vi "GetVariableIDs_Example.vi"(8 "Fehler (Eingang, kein Fehler)":errorcluster) -> (0 "Fehler (Ausgang)":errorcluster, 3 "VariableArray out":T1)   [LabVIEW 2016]
uses:
  VariableArray.ctl
  VariableInfo.ctl
  girpcutil_params.ctl
panel:
  out "State":string
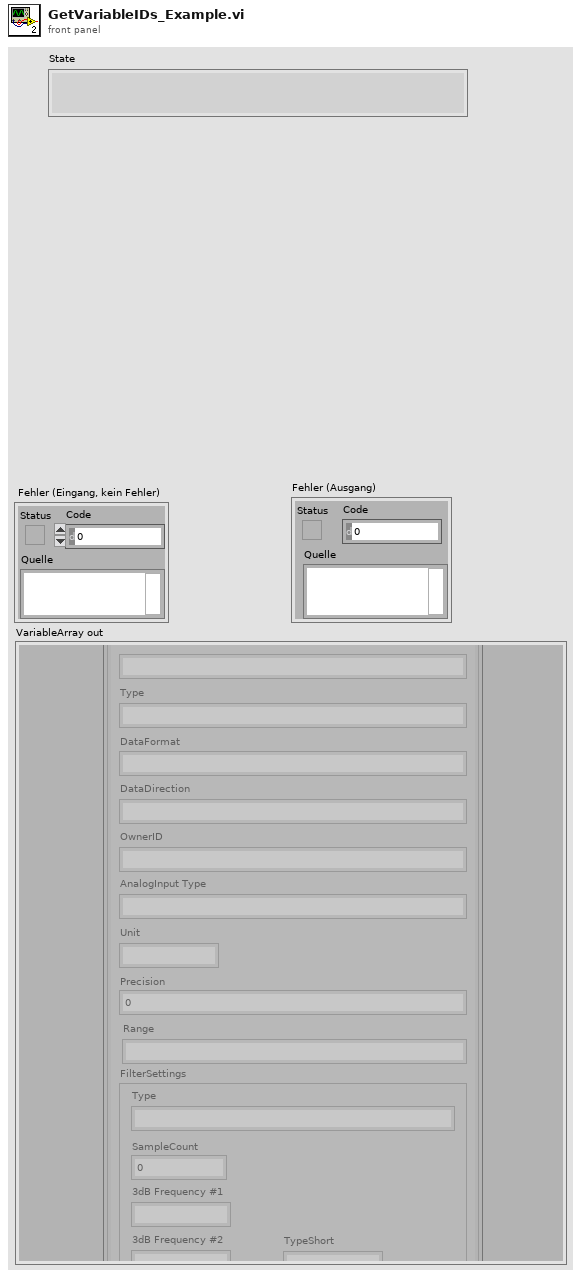
[diagram p1: front panel]
types:
  T1 = typedef "VariableArray.ctl" = cluster{"Array":T2[]}
  T2 = typedef "VariableInfo.ctl" = cluster{"Name":string, "ID":string, "Type":string, "DataFormat":string, "DataDirection":string, "OwnerID":string, "AnalogInput Type":string, "Unit":string, "Precision":dbl, "Range":string, "FilterSettings":cluster{"Type":string, "SampleCount":i64, "3dB Frequency #1":string, "3dB Frequency #2":string, "TypeShort":string}}
  T3 = typedef "girpcutil_params.ctl" = cluster{"ConnectionHandle":i32, "DLL-Handle":cluster{"DLL Path":path, "Is32Bit":bool}}
  T4 = enum16{"Bool", "Snippet", "Struct", "Int64", "Int32", "Float", "Double", "String"}
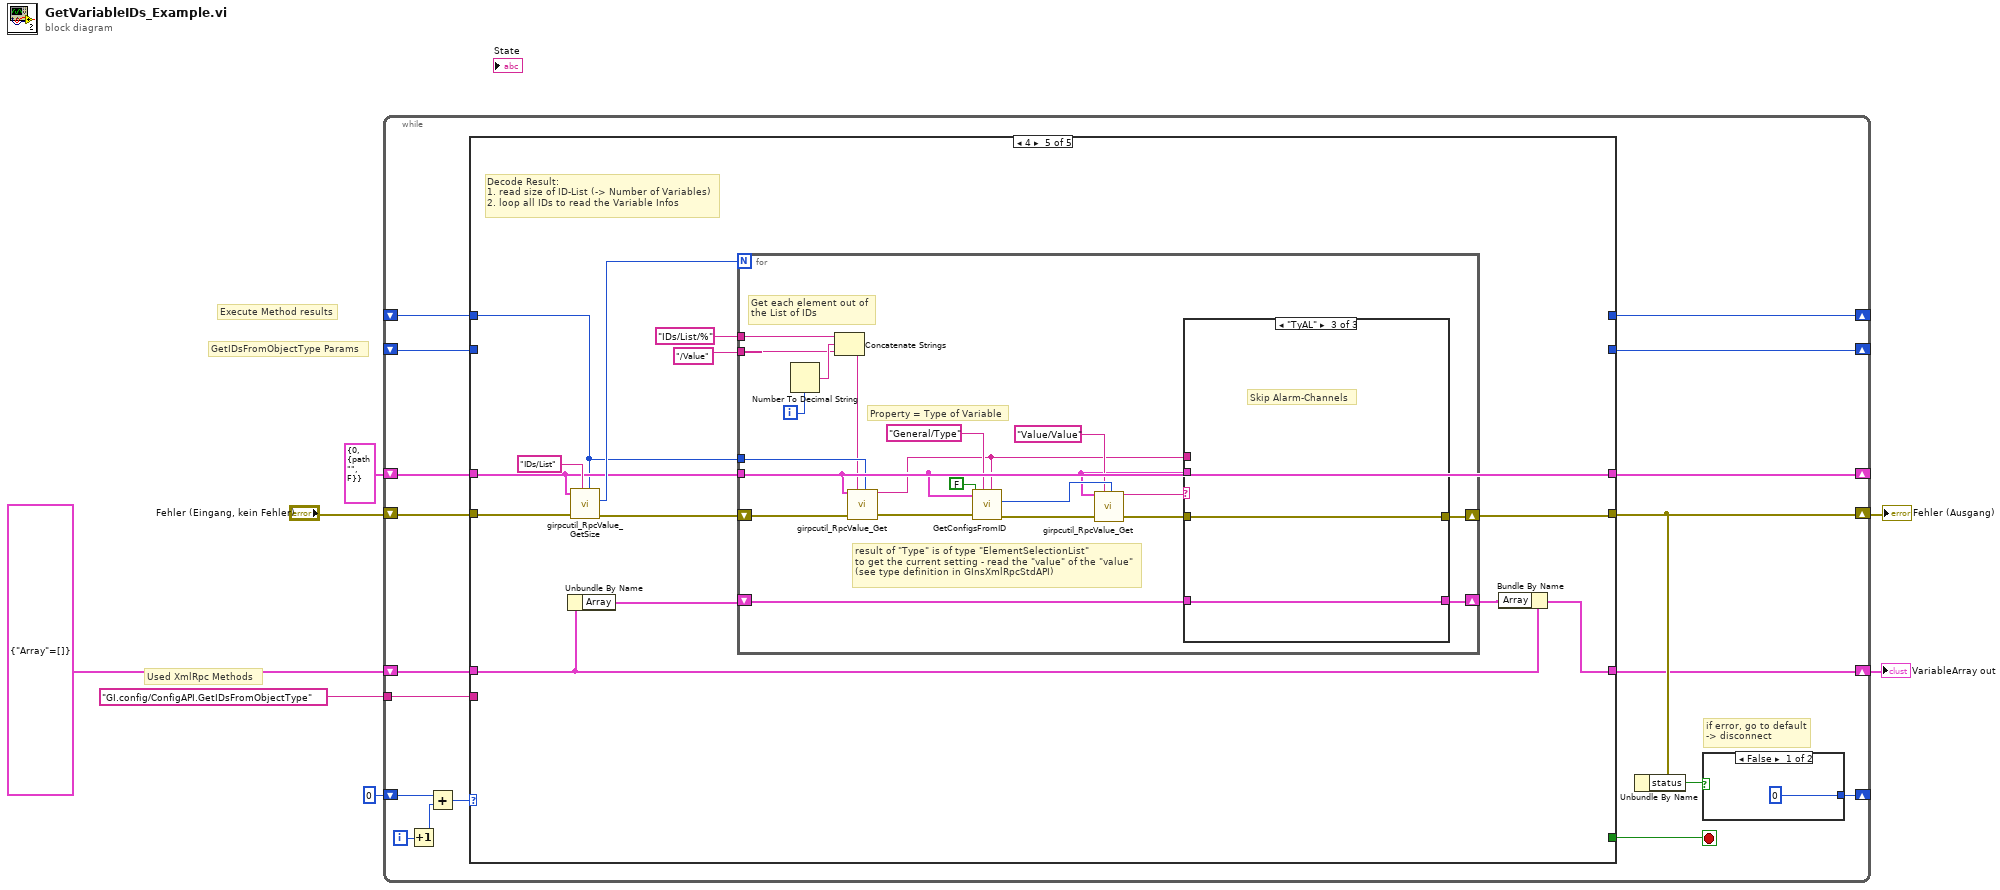
[diagram p0: block diagram]
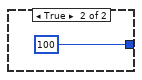
[diagram p2: hidden frame]
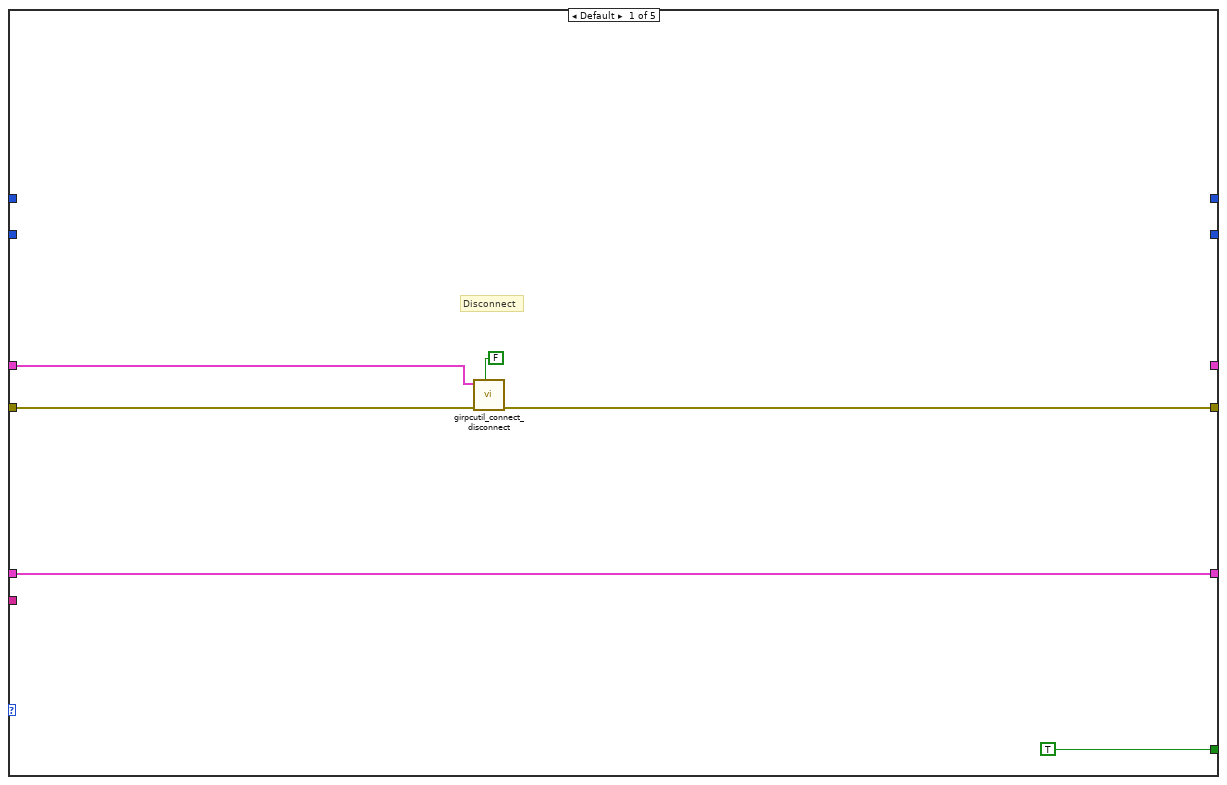
[diagram p3: hidden frame]
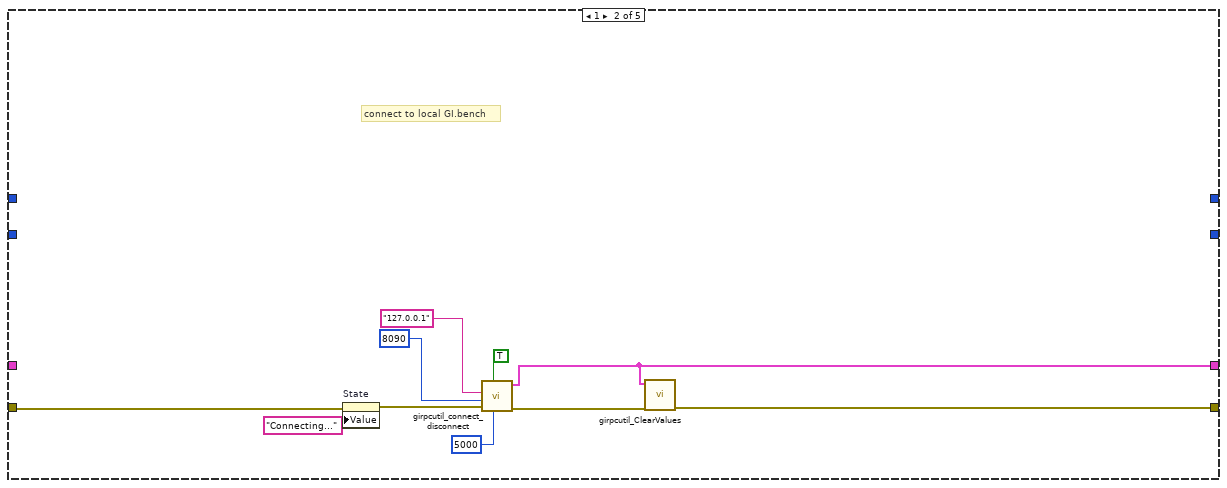
[diagram p4: hidden frame]
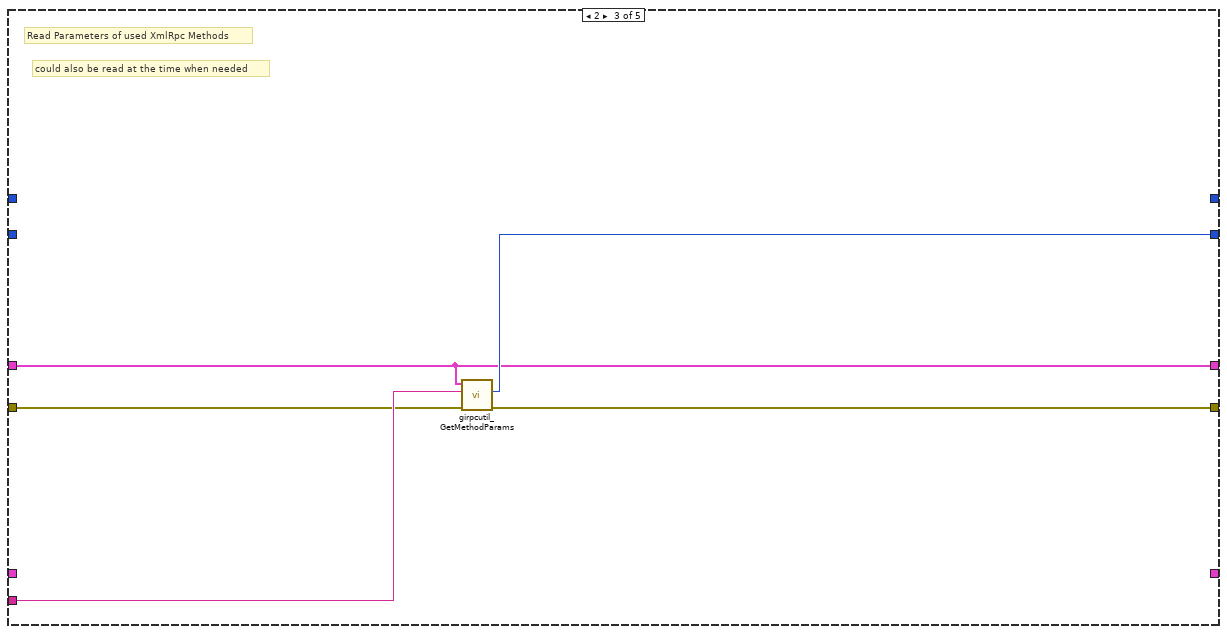
[diagram p5: hidden frame]
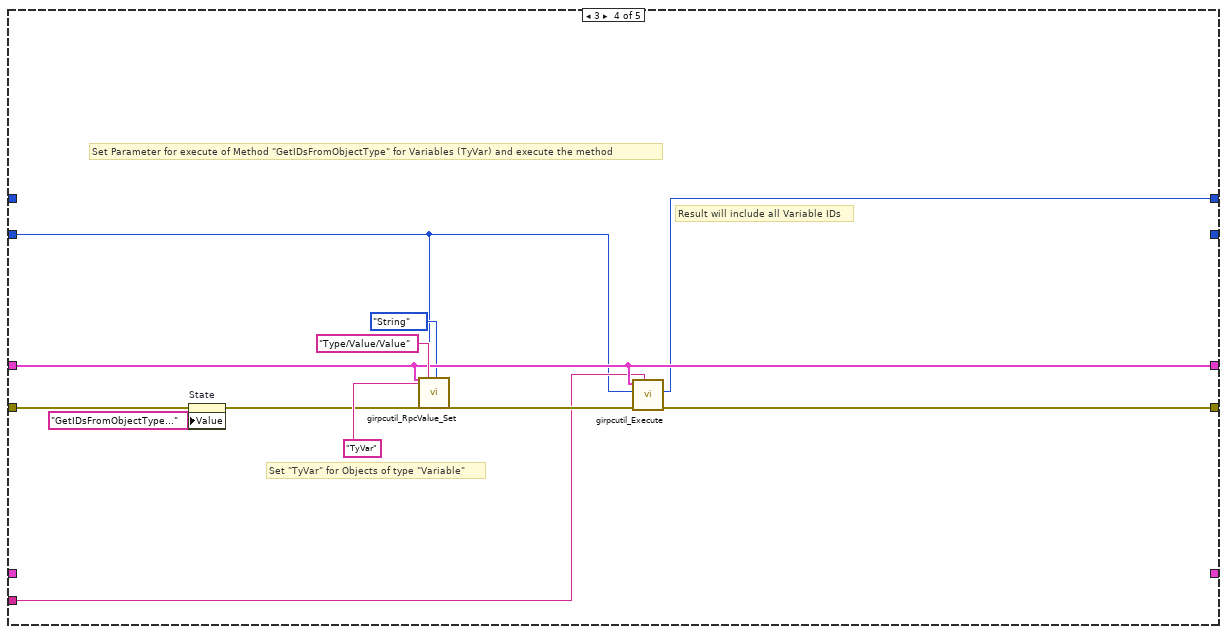
[diagram p6: hidden frame]
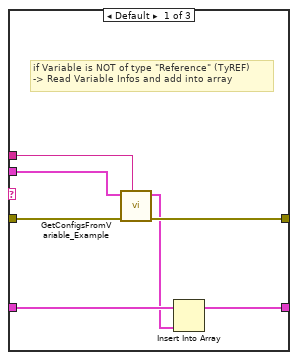
[diagram p7: hidden frame]
diagram:
  # "Execute Method results"
  # "GetIDsFromObjectType Params"
  # "Used XmlRpc Methods"
  n1 = while {
    shift-right: [w19] -> w6
    shift-left: "Fehler (Eingang, kein Fehler)" -> [w24]
    tunnel: "GI.config/ConfigAPI.GetIDsFromObjectType" ("methodName") -> [w23]
    shift-right: [w22] -> _
    shift-left: T3 {"ConnectionHandle"=0, "DLL-Handle"={"DLL Path"=path "", "Is32Bit"=FALSE}} ("girpcutil_params 2") -> [w21]
    shift-right: [w20] -> _
    shift-left: _ -> [w18]
    shift-right: [w12] -> _
    shift-left: 0 -> [w13]
    shift-right: [w11] -> _
    shift-left: _ -> [w10]
    shift-right: [w9] -> w3
    shift-left: T1 {"Array"=[]} ("VariableArray") -> [w8]
    i -> [w25]
    stop <- w17 stop-if-true
    # "if error, go to default\n-> disconnect"
    n2 = Increment(x=w25) -> (x+1=w15:i32)
    n3 = Add(x=w13, y=w15) -> (x+y=w14:i32)
    n4 = case shown="4" w14 {
      tunnel: [TRUE _ _ _ _] -> w17
      tunnel: w24 -> [w32 w34 w45 w54 w73]
      tunnel: [w31 w38 w46 w57 w69] -> w19
      tunnel: w23 -> [_ _ w48 w51 _]
      tunnel: [_ w37 w44 w56 w68] -> w22
      tunnel: w21 -> [w30 _ w44 w56 w68]
      tunnel: [_ _ w47 _ _] -> w20
      tunnel: w18 -> [_ _ _ w50 _]
      tunnel: [_ _ _ w49 _] -> w11
      tunnel: w10 -> [_ _ _ _ w67]
      tunnel: [w28 _ _ _ w63] -> w9
      tunnel: w8 -> [w28 _ _ _ w61]
      frame Default {
        # "Disconnect"
        n5 = call "girpcutil_connect_disconnect.vi"("Connect"=FALSE, "Fehler (Eingang, kein Fehler)"=w32, "girpcutil_params"=w30) -> ("Fehler (Ausgang)"=w31:errorcluster)  [unwired: 7 in, 1 out]
      }
      frame 1 {
        # "connect to local GI.bench"
        n6 = property on="State" class="Str"(error in=w34, "Value"="Connecting..." ("State")) -> (error out=w36:errorcluster)  [unwired: 1 in, 1 out]
        n7 = call "girpcutil_connect_disconnect.vi"("timeout"=u32 5000, "Connect"=TRUE, "Fehler (Eingang, kein Fehler)"=w36, "port"=u32 8090, "host"="127.0.0.1") -> ("Fehler (Ausgang)"=w39:errorcluster, "girpcutil_params 2"=w37:T3)  [unwired: 5 in]
        n8 = call "girpcutil_ClearValues.vi"("Fehler (Eingang, kein Fehler)"=w39, "girpcutil_params"=w37) -> ("error IO"=w38:errorcluster)  [unwired: 9 in]
      }
      frame 2 {
        # "could also be read at the time when needed"
        # "Read Parameters of used XmlRpc Methods"
        n9 = call "girpcutil_GetMethodParams.vi"("Fehler (Eingang, kein Fehler)"=w45, "methodName"=w48, "girpcutil_params"=w44) -> ("Fehler (Ausgang)"=w46:errorcluster, "param handle out"=w47:i32)  [unwired: 7 in]
      }
      frame 3 {
        # "Result will include all Variable IDs"
        # "Set \"TyVar\" for Objects of type \"Variable\""
        # "Set Parameter for execute of Method \"GetIDsFromObjectType\" for Variables (TyVar) and execute the method"
        n10 = property on="State" class="Str"(error in=w54, "Value"="GetIDsFromObjectType..." ("State")) -> (error out=w53:errorcluster)  [unwired: 1 in, 1 out]
        n11 = call "girpcutil_RpcValue_Set.vi"("girpcutil_params"=w56, "StringValue or Snippet"="TyVar", "Fehler (Eingang, kein Fehler)"=w53, "MemberName"="Type/Value/Value", "param handle"=w50, "DataType"=T4."String") -> ("Fehler (Ausgang)"=w58:errorcluster)  [unwired: 21 in]
        n12 = call "girpcutil_Execute.vi"("methodName"=w51, "Fehler (Eingang, kein Fehler)"=w58, "params"=w50, "girpcutil_params"=w56) -> ("Fehler (Ausgang)"=w57:errorcluster, "results"=w49:i32)  [unwired: 6 in]
      }
      frame 4 {
        # "Decode Result:\n1. read size of ID-List (-> Number of Variables)\n2. loop all IDs to read the Variable Infos"
        n13 = Unbundle By Name(w61) -> ("Array"=w62:T2[])
        n14 = call "girpcutil_RpcValue_GetSize.vi"("param handle"=w67, "member"="IDs/List", "Fehler (Eingang, kein Fehler)"=w73, "girpcutil_params"=w68) -> ("Fehler (Ausgang)"=w70:errorcluster, "size"=w71:u64)  [unwired: 6 in]
        n15 = for {
          N: w71 -> [_]
          shift-right: [w80] -> w69
          shift-left: w70 -> [w93]
          tunnel: w68 -> [w79]
          tunnel: w67 -> [w92]
          tunnel: "IDs/List/%" ("member") -> [w90]
          tunnel: "/Value" ("member") -> [w88]
          shift-right: [w77] -> w64
          shift-left: w62 -> [w78]
          i -> [w91]
          # "Get each element out of \nthe List of IDs"
          # "Property = Type of Variable"
          # "result of \"Type\" is of type \"ElementSelectionList\"\nto get the current setting - read the \"value\" of the \"value\"\n(see type definition in GInsXmlRpcStdAPI)"
          n16 = Number To Decimal String(number=w91) -> (decimal integer string=w89:string)  [unwired: 1 in]
          n17 = Concatenate Strings(w90, w89, w88) -> (w87:string)
          n18 = call "girpcutil_RpcValue_Get.vi"("girpcutil_params"=w79, "Fehler (Eingang, kein Fehler)"=w93, "member"=w87, "value"=w92) -> ("StringResult"=w75:string, "Fehler (Ausgang)"=w86:errorcluster)  [unwired: 19 in, 3 out]
          n19 = call "GetConfigsFromID.vi"("ID"=w75, "PropertyName"="General/Type", "Fehler (Eingang, kein Fehler)"=w86, "WithOptions"=FALSE, "girpcutil_params"=w79) -> ("Fehler (Ausgang)"=w84:errorcluster, "StructResult"=w83:i32)  [unwired: 5 in]
          n20 = call "girpcutil_RpcValue_Get.vi"("girpcutil_params"=w79, "Fehler (Eingang, kein Fehler)"=w84, "member"="Value/Value", "value"=w83) -> ("StringResult"=w76:string, "Fehler (Ausgang)"=w81:errorcluster)  [unwired: 19 in, 3 out]
          n21 = case shown="\"TyAL\"" w76 {
            tunnel: w81 -> [w98 w102 w104]
            tunnel: [w97 w102 w104] -> w80
            tunnel: w75 -> [w94 _ _]
            tunnel: w79 -> [w95 _ _]
            tunnel: w78 -> [w100 w101 w103]
            tunnel: [w99 w101 w103] -> w77
            frame Default {
              # "if Variable is NOT of type \"Reference\" (TyREF)\n-> Read Variable Infos and add into array"
              n22 = call "GetConfigsFromVariable_Example.vi"("ID"=w94, "Fehler (Eingang, kein Fehler)"=w98, "girpcutil_params"=w95) -> ("Fehler (Ausgang)"=w97:errorcluster, "VariableInfo out"=w96:T2)  [unwired: 7 in]
              n23 = Insert Into Array(array=w100, new element=w96) -> (w99:T2[])  [unwired: 1 in]
            }
            frame "TyREF" {
              # "Skip Reference-Variables"
            }
            frame "TyAL" {
              # "Skip Alarm-Channels"
            }
          }
        }
        n24 = Bundle By Name(cluster=w61, "Array"=w64) -> (w63:T1)
      }
    }
    n25 = Unbundle By Name(w19) -> ("status"=w16:bool)
    n26 = case shown="False" w16 {
      tunnel: [0 100] -> w12
      frame False {
      }
      frame True {
      }
    }
  }
  "Fehler (Ausgang)" <- w6
  "VariableArray out" <- w3
